vi "Launcher.vi"() -> ()   [LabVIEW 2014, in "Camera Display.lvlib"]
uses:
  Camera Display.lvlib
  Launch IMAQ Display/Camera Display.lvclass
  <vilib>/ActorFramework/Actor/Actor.lvclass
panel:
  out "error out":errorcluster
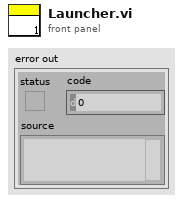
[diagram p1: front panel]
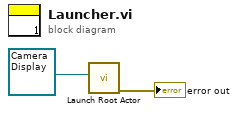
[diagram p0: block diagram]
diagram:
  n1 = call <vilib>:"Launch Root Actor.vi"("Actor"=refnum<class "Camera Display.lvclass"> refnum ("Launch IMAQ Display.lvlib:Launch IMAQ Display.lvclass")) -> ("error out"=→"error out":errorcluster)  [unwired: 9 in, 1 out]
